vi "Hysteresis-LookForCovarianceMaximum.vi"(9 "size":i32, 10 "Cluster filtered":cluster{dbl, i32, i32}[](array[cluster]), 11 "Covariance Values (1D)":dbl[](array[numeric])) -> (2 "BWD/FWD":cluster{"bwd column":i32[], "fwd column":i32[]}, 3 "Values":dbl[](array[numeric]))   [LabVIEW 2016]
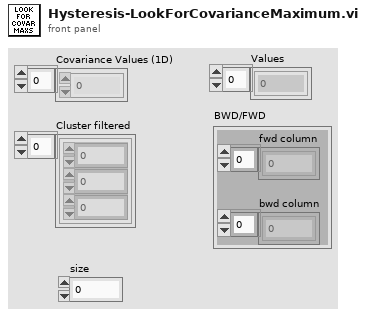
[diagram p1: front panel]
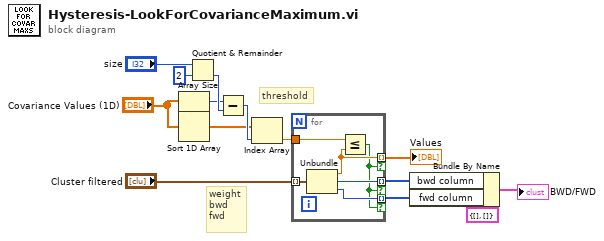
[diagram p0: block diagram]
diagram:
  # "weight\nbwd\nfwd"
  # "threshold"
  n1 = Array Size(array="Covariance Values (1D)") -> (size(s)=w8:i32)
  n2 = Sort 1D Array(array="Covariance Values (1D)") -> (sorted array=w7:dbl[])
  n3 = Quotient & Remainder(x="size", y=2) -> (floor(x/y)=w12:i32)  [unwired: 1 out]
  n4 = Subtract(x=w8, y=w12) -> (x-y=w11:i32)
  n5 = Index Array(array=w7, index=w11) -> (element=w10:dbl)
  n6 = for {
    tunnel: "Cluster filtered" -> [w20] mode=indexing
    tunnel: w10 -> [w19]
    tunnel: [w18] -> w14 mode=indexing if=w15
    tunnel: [w17] -> w4 mode=indexing if=w15
    tunnel: [w16] -> w3 mode=indexing if=w15
    n7 = Unbundle(w20) -> (w18:dbl, w17:i32, w16:i32)
    n8 = Less Or Equal?(x=w19, y=w18) -> (x <= y?=w15:bool)
  }
  "Values" <- w14
  n9 = Bundle By Name(cluster=cluster{"bwd column":i32[], "fwd column":i32[]} {"bwd column"=[], "fwd column"=[]} ("Cluster"), "bwd column"=w4, "fwd column"=w3) -> (→"BWD/FWD":cluster{"bwd column":i32[], "fwd column":i32[]})
